vi "get_discont_step_size_float.vi"(9 "current pixel (iteration)":i32, 11 "current row in image":dbl[](array[numeric])) -> (3 "step_size":dbl)   [LabVIEW 2011]
doc: "Calculates the step size between the two pixels of a discontinuity. The step size is calulated by the difference between the two pixels plus an average slope, calculate as the average slope before and after the discontinuity."
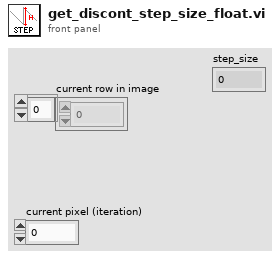
[diagram p1: front panel]
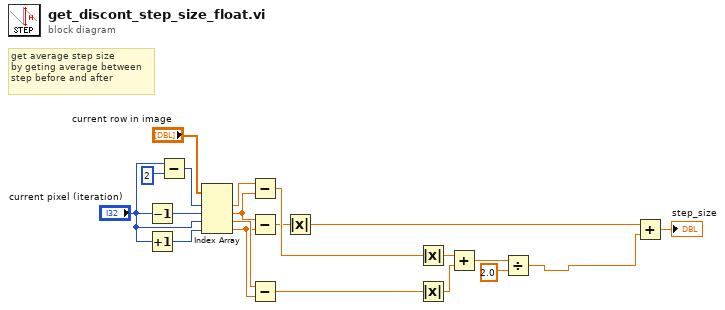
[diagram p0: block diagram]
diagram:
  # "get average step size\nby geting average between\nstep before and after"
  n1 = Decrement(x="current pixel (iteration)") -> (x-1=w11:i32)
  n2 = Increment(x="current pixel (iteration)") -> (x+1=w10:i32)
  n3 = Subtract(x="current pixel (iteration)", y=2) -> (x-y=w12:i32)
  n4 = Index Array(array="current row in image", index #1=w12, index #2=w11, index #3="current pixel (iteration)", index #4=w10) -> (element #1=w8:dbl, element #2=w6:dbl, element #3=w7:dbl, element #4=w5:dbl)
  n5 = Subtract(x=w8, y=w6) -> (x-y=w16:dbl)
  n6 = Subtract(x=w6, y=w5) -> (x-y=w4:dbl)
  n7 = Subtract(x=w7, y=w5) -> (x-y=w15:dbl)
  n8 = Absolute Value(x=w4) -> (abs(x)=w3:dbl)
  n9 = Absolute Value(x=w16) -> (abs(x)=w17:dbl)
  n10 = Absolute Value(x=w15) -> (abs(x)=w18:dbl)
  n11 = Add(x=w17, y=w18) -> (x+y=w19:dbl)
  n12 = Divide(x=w19, y=2.0) -> (x/y=w1:dbl)
  n13 = Add(x=w3, y=w1) -> (x+y=→"step_size":dbl)
